vi "gfitsio-check-valid-refnum.vi"(4 "gftis refnum":T1) -> (1 "invalid refnum?":bool)   [LabVIEW 2023, in "gfitsio.lvlib"]
doc: "Returns TRUE if <B>gftis refnum</B> is invalid. Use this function to make sure a reference to a file still resides in system memory and was not closed."
uses:
  gfitsio.lvlib
  gfitsio.dll
  gfitsio-refnum.ctl
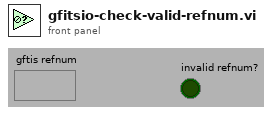
[diagram p1: front panel]
types:
  T1 = typedef "gfitsio.lvlib/gfitsio-refnum.ctl" = refnum<k1>
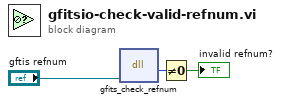
[diagram p0: block diagram]
diagram:
  n1 = dll-call lib="gfitsio.dll" fn="gfits_check_refnum"("refnum"="gftis refnum") -> (w3:i32)  [unwired: 4 in, 2 out]
  n2 = Not Equal To 0?(x=w3) -> (x != 0?=→"invalid refnum?":bool)
